vi "Run.vi"(8 "error in (no error)":errorcluster, 9 "s on last turn":dbl, 10 "Maze (0: Empty, -1: Enemy. >0: Teammate":i32[][](array[numeric]), 11 "Wanderer in":refnum<class "Wanderer.lvclass">) -> (0 "error out":errorcluster, 1 "Direction":T1, 2 "Action":T2, 3 "Wanderer out":refnum<class "Wanderer.lvclass">, 4 "Replicated":refnum<class "Square.lvclass">)   [LabVIEW 2015, in "Wanderer.lvclass"]
uses:
  Wanderer.lvclass
  Type Defs/Action Enum.ctl
  Type Defs/Direction Enum.ctl
  Square/Square.lvclass
  Carl/Coward/Coward.lvclass
  Wanderer.lvclass/Wanderer.ctl
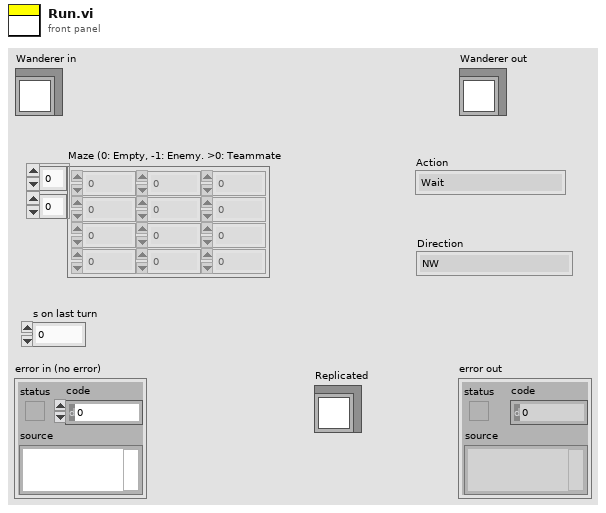
[diagram p1: front panel]
types:
  T1 = typedef "Square.lvclass/Direction Enum.ctl" = enum16{"NW", "N", "NE", "E", "SE", "S", "SW", "W"}
  T2 = typedef "Square.lvclass/Action Enum.ctl" = enum16{"Wait", "Move", "Attack", "Replicate"}
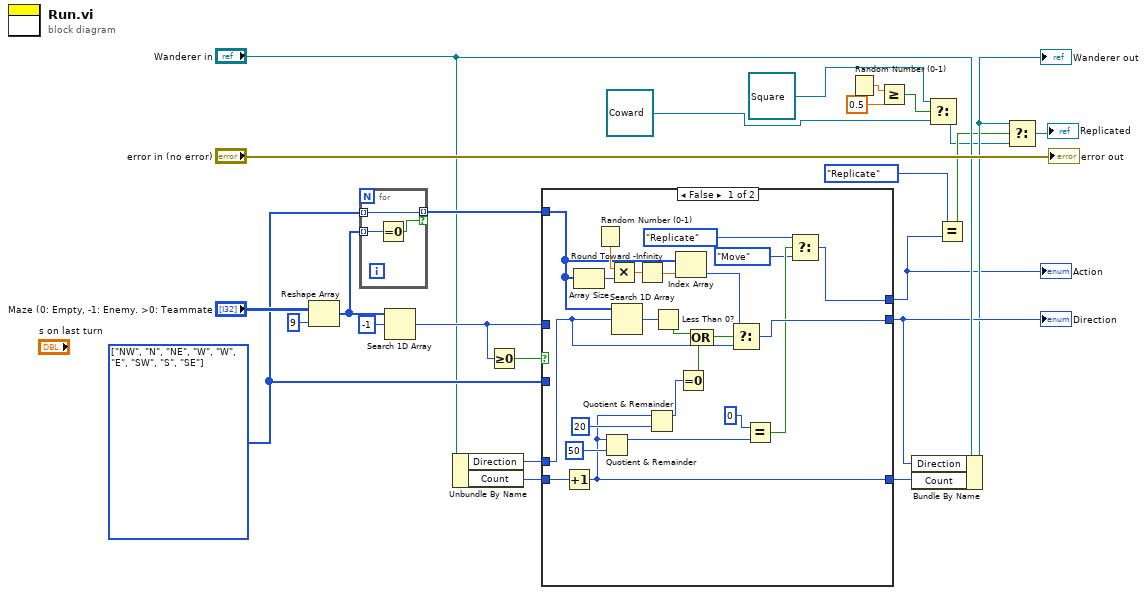
[diagram p0: block diagram]
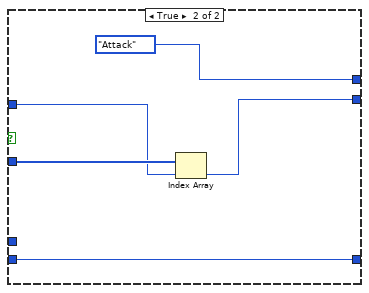
[diagram p2: hidden frame]
diagram:
  w18 = T1[] [enum."NW", enum."N", enum."NE", enum."W", enum."W", enum."E", enum."SW", enum."S", enum."SE"] items=["NW", "N", "NE", "E", "SE", "S", "SW", "W"]
  n1 = Reshape Array("Maze (0: Empty, -1: Enemy. >0: Teammate", 9 ("dimension size")) -> (w22:i32[])
  n2 = for {
    tunnel: w22 -> [w28] mode=indexing
    tunnel: w18 -> [w27] mode=indexing
    tunnel: [w27] -> w20 mode=indexing if=w26
    n3 = Equal To 0?(x=w28) -> (x = 0?=w26:bool)
  }
  n4 = Search 1D Array(1D array=w22, element=-1) -> (index of element=w21:i32)  [unwired: 1 in]
  n5 = Unbundle By Name("Wanderer in") -> ("Direction"=w13:T1, "Count"=w15:i32)
  n6 = Greater Or Equal To 0?(x=w21) -> (x >= 0?=w23:bool)
  n7 = case shown="False" w23 {
    tunnel: [w49 Action_Enum."Attack" ("Action")] -> w10
    tunnel: w21 -> [_ w55]
    tunnel: w18 -> [_ w56]
    tunnel: [w39 w54] -> w12
    tunnel: w20 -> [w37 _]
    tunnel: w15 -> [w31 w52]
    tunnel: [w30 w52] -> w14
    tunnel: w13 -> [w29 _]
    frame False {
      n8 = Increment(x=w31) -> (x+1=w30:i32)
      n9 = Array Size(array=w37) -> (size(s)=w47:i32)
      n10 = Random Number (0-1)() -> (number: 0 to 1=w48:dbl)
      n11 = Quotient & Remainder(x=w30, y=50 ("dimension size")) -> (x-y*floor(x/y)=w44:i32)  [unwired: 1 out]
      n12 = Multiply(x=w48, y=w47) -> (x*y=w38:dbl)
      n13 = Search 1D Array(1D array=w37, element=w29) -> (index of element=w46:i32)  [unwired: 1 in]
      n14 = Round Toward -Infinity(1:w38) -> (0:w36:dbl)
      n15 = Quotient & Remainder(x=w30, y=20 ("dimension size")) -> (x-y*floor(x/y)=w42:i32)  [unwired: 1 out]
      n16 = Less Than 0?(x=w46) -> (x < 0?=w45:bool)
      n17 = Index Array(array=w37, index=w36) -> (element=w35:T1)
      n18 = Equal To 0?(x=w42) -> (x = 0?=w41:bool)
      n19 = Compound Arithmetic op=OR(w45, w41) -> (w40:bool)
      n20 = Select(t=w35, s=w40, f=w29) -> (s? t:f=w39:T1)
      n21 = Equal?(x=0, y=w44) -> (x = y?=w34:bool)
      n22 = Select(t=Action_Enum."Replicate" ("Action"), s=w34, f=Action_Enum."Move" ("Action")) -> (s? t:f=w49:T2)
    }
    frame True {
      n23 = Index Array(array=w56, index=w55) -> (element=w54:T1)
    }
  }
  "Action" <- w10
  "Direction" <- w12
  n24 = Random Number (0-1)() -> (number: 0 to 1=w6:dbl)
  n25 = Greater Or Equal?(x=w6, y=0.5) -> (x >= y?=w4:bool)
  n26 = Bundle By Name(cluster="Wanderer in", "Direction"=w12, "Count"=w14) -> (w11:refnum<class "Wanderer.lvclass">)
  "Wanderer out" <- w11
  n27 = Select(t=refnum<class "Square.lvclass"> refnum ("Runner.lvclass"), s=w4, f=refnum<class "Coward.lvclass"> refnum ("Coward.lvclass")) -> (s? t:f=w2:refnum<class "Square.lvclass">)
  n28 = Equal?(x=Action_Enum."Replicate", y=w10) -> (x = y?=w9:bool)
  n29 = Select(t=w11, s=w9, f=w2) -> (s? t:f=→"Replicated":refnum<class "Square.lvclass">)
  "error out" <- "error in (no error)"
